vi "Fix Relocated Aliases.vi"(8 "error in (no error)":errorcluster, 10 "Outdated Dependent Modules":cluster{"Old Path":string, "New Path":string}[](array[cluster]), 11 "Endpoint Aliases Ref in":T1 format="%.0x") -> (0 "error out":errorcluster, 3 "Endpoint Aliases Ref out":T1 format="%.0x")   [LabVIEW 2017, in "Routing and Faulting Scripting.lvlib"]
uses:
  <vilib>/NI Veristand/Custom Device API/Custom Device Item Ref.ctl
  Routing and Faulting Scripting.lvlib
  System Explorer/Routing and Faulting System Explorer.lvlib
  <vilib>/NI Veristand/Custom Device API/Custom Device API.lvlib
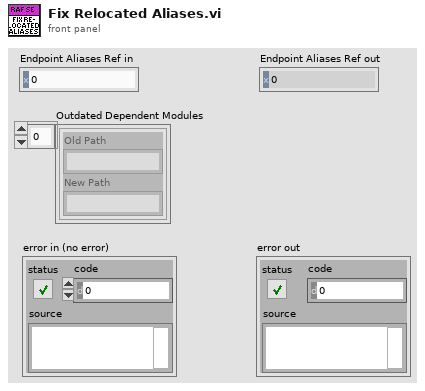
[diagram p1: front panel]
types:
  T1 = typedef "Custom Device API.lvlib/Custom Device Item Ref.ctl" = u64
  T2 = typedef "Routing and Faulting Shared.lvlib/Alias Mapping.ctl" = cluster{"Endpoint":string, "Alias":string}
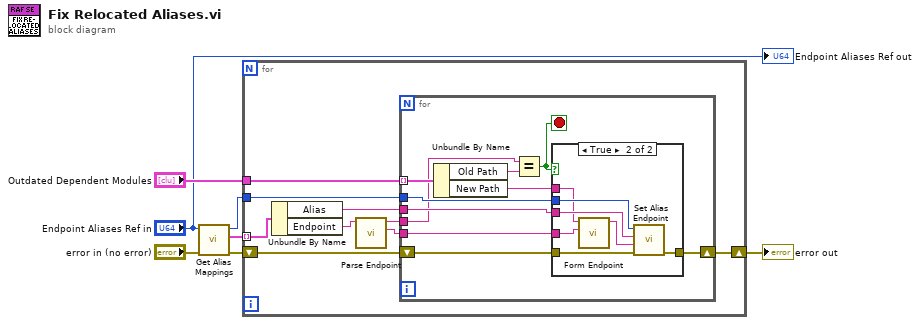
[diagram p0: block diagram]
diagram:
  n1 = call "Get Alias Mappings.vi"("error in (no error)"="error in (no error)", "Endpoint Aliases Ref in"="Endpoint Aliases Ref in") -> ("error out"=w4:errorcluster, "Alias Mappings"=w1:T2[], "Endpoint Aliases Ref out"=w2:T1)  [unwired: 7 in]
  n2 = for {
    tunnel: w1 -> [w16] mode=indexing
    tunnel: "Outdated Dependent Modules" -> [w15]
    shift-right: [w12] -> w5
    shift-left: w4 -> [w13]
    tunnel: w2 -> [w14]
    n3 = Unbundle By Name(w16) -> ("Alias"=w11:string, "Endpoint"=w10:string)
    n4 = call "Parse Endpoint.vi"("Resource/Endpoint"=w10) -> ("Endpoint"=w9:string, "Resource"=w8:string)  [unwired: 9 in]
    n5 = for {
      tunnel: w15 -> [w26] mode=indexing
      shift-right: [w21] -> w12
      shift-left: w13 -> [w22]
      tunnel: w14 -> [w23]
      tunnel: w11 -> [w20]
      tunnel: w9 -> [w17]
      tunnel: w8 -> [w19]
      stop <- w24 stop-if-true
      n6 = Unbundle By Name(w26) -> ("Old Path"=w25:string, "New Path"=w18:string)
      n7 = Equal?(x=w19, y=w25) -> (x = y?=w24:bool)
      n8 = case shown="True" w24 {
        tunnel: w23 -> [_ w34]
        tunnel: w22 -> [w27 w33]
        tunnel: [w27 w32] -> w21
        tunnel: w20 -> [_ w31]
        tunnel: w18 -> [_ w29]
        tunnel: w17 -> [_ w28]
        frame False {
        }
        frame True {
          n9 = call "Form Endpoint.vi"("Endpoint"=w28, "Resource"=w29) -> ("Resource/Endpoint"=w30:string)  [unwired: 9 in]
          n10 = call "Set Alias Endpoint.vi"("error in (no error)"=w33, "New Endpoint"=w30, "Alias"=w31, "Endpoint Aliases Ref in"=w34) -> ("error out"=w32:errorcluster)  [unwired: 6 in, 1 out]
        }
      }
    }
  }
  "error out" <- w5
  "Endpoint Aliases Ref out" <- "Endpoint Aliases Ref in"
